vi "Modbus Master Example.vi"() -> ()   [LabVIEW 2013, in "Modbus Library - Advance.lvlib"]
doc: "An example of the modbus master functionality."
uses:
  Modbus Library - Advance.lvlib
  API/Wrapper/API Main.lvlib
  Master Function Definition/Read Device ID code.ctl
  Data Model/Device Data Model.lvclass
  API/Master/Modbus Master.lvclass
  API/Wrapper/Create TCP Master.vi
panel:
  in  "unit ID":u8=1
  in  "Stop Button":bool
  in  "Port":u16=502
  in  "Set Holding Registers":bool
  in  "Set Coils":bool
  in  "Fetch Discrete Inputs":bool
  in  "Fetch Input Registers":bool
  in  "Fetch Basic Objects":bool
  out "Basic Objects":string[](array[string])
  out "Status":string
  in  "Disconnect":bool
  in  "Connect":bool
  in  "Holding Registers":u16[](array[numeric])=[0, 0, 0, 0, 0, 0, 0, 0]
  out "Input Registers":u16[](array[numeric])
  in  "Coils":bool[](array[boolean])=[FALSE, FALSE, FALSE, FALSE, FALSE, FALSE, FALSE, FALSE]
  out "Discrete Inputs":bool[](array[boolean])
  in  "Slave Address":string="localhost"
  # "Coils are the boolean outputs of a modbus device. This example allows you to set the first 8 outputs."
  # "Holding Registers are the integer outputs of a modbus device. This example allows you to set the first 8 outputs."
  # "Modbus devices can also store objects in their memory, which are variable length strings. This example requests the basic level of objects."
  # "Discrete inputs are the boolean inputs of a modbus device. This example allows you to read the first 8 inputs."
  # "Input Registers are the integer inputs of a modbus device. This example allows you to read the first 8 inputs."
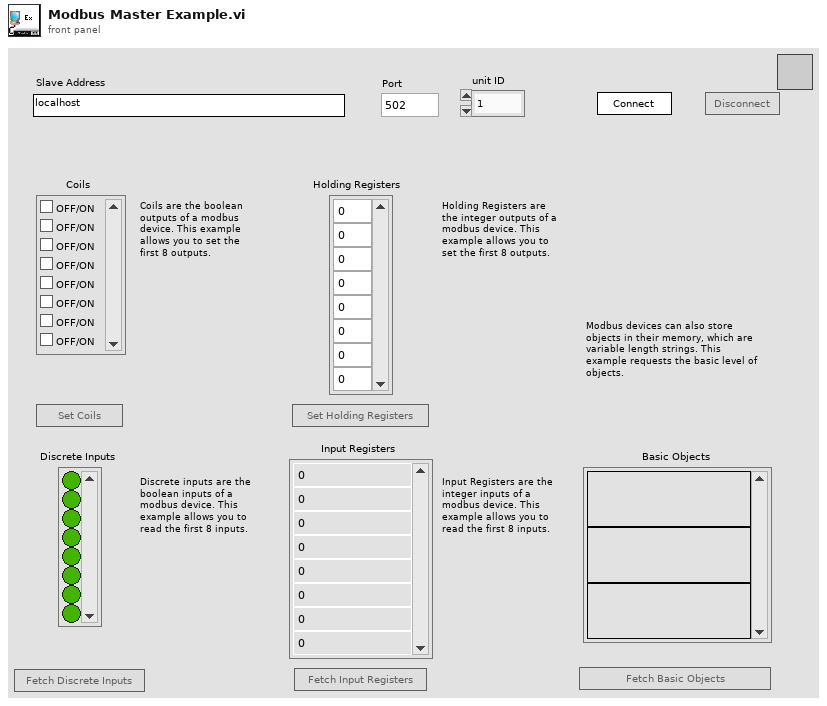
[diagram p1: front panel]
types:
  T1 = enum8{"Enabled", "Disabled", "Disabled and Grayed Out"}
  T2 = typedef "Modbus Library - Advance.lvlib/Device Data Model.lvclass/Read Device ID code.ctl" = enum8{"Read Basic", "Read Regular", "Read Extended", "Read Specific"}
  T3 = typedef "Modbus Library - Advance.lvlib/Device Data Model.lvclass/Identification Parameters.ctl" = cluster{"Object ID":u8, "Value":string}
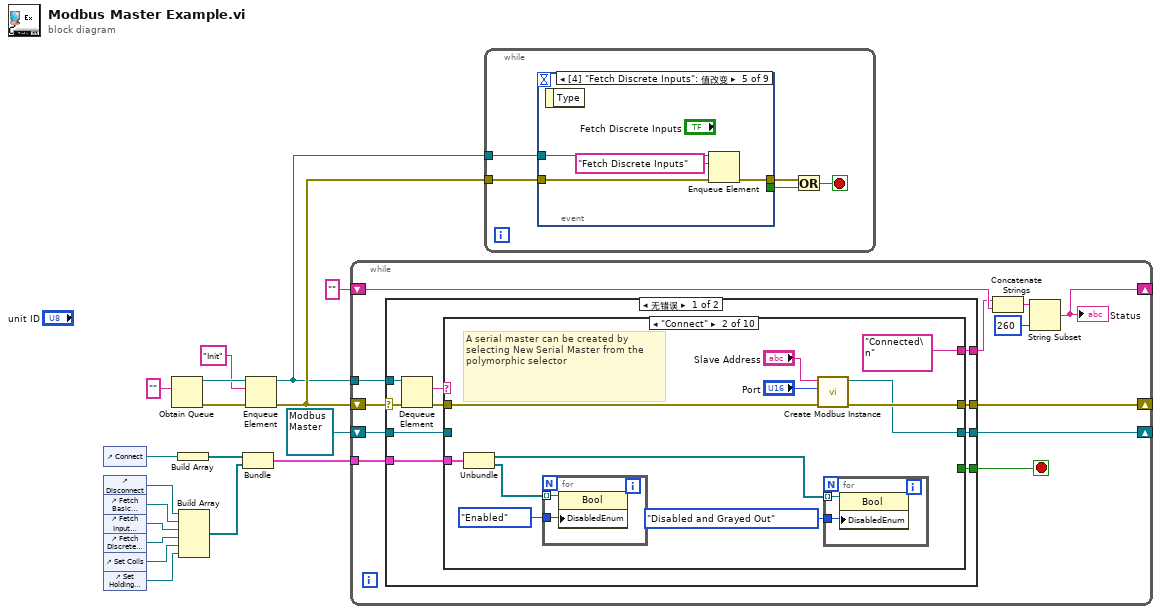
[diagram p0: block diagram]
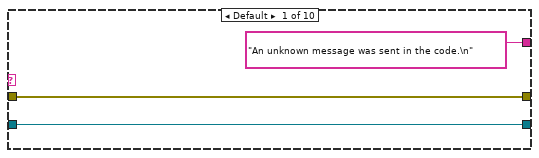
[diagram p2: hidden frame]
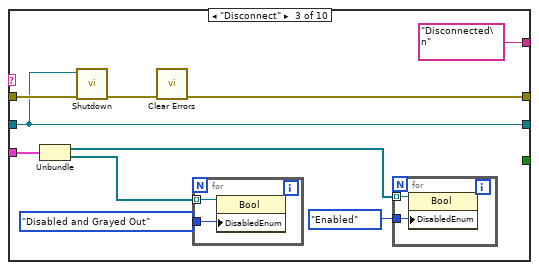
[diagram p3: hidden frame]
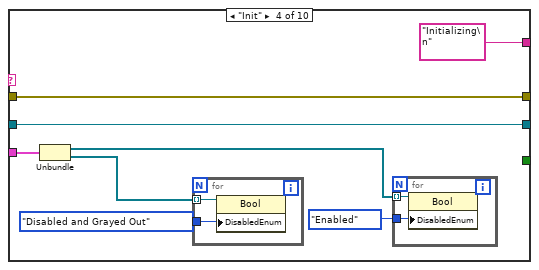
[diagram p4: hidden frame]
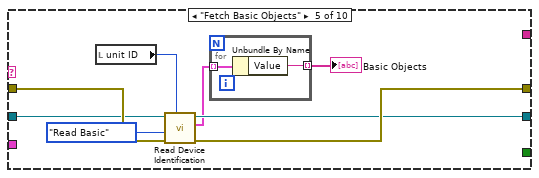
[diagram p5: hidden frame]
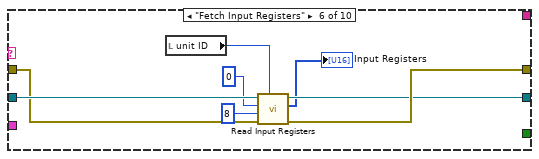
[diagram p6: hidden frame]
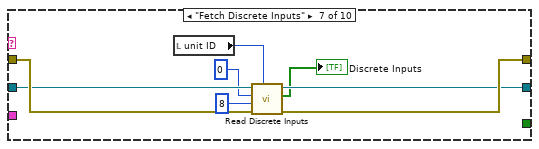
[diagram p7: hidden frame]
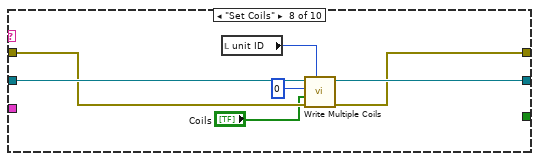
[diagram p8: hidden frame]
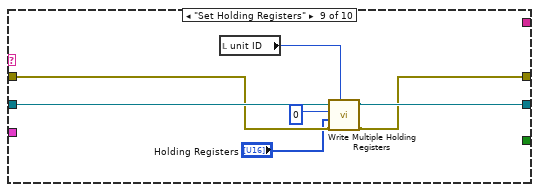
[diagram p9: hidden frame]
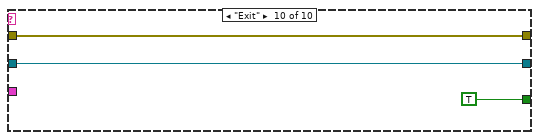
[diagram p10: hidden frame]
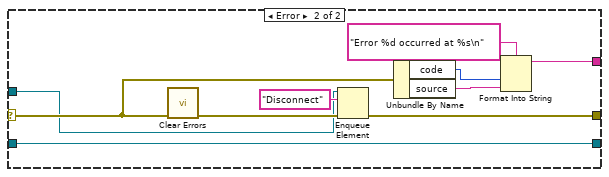
[diagram p11: hidden frame]
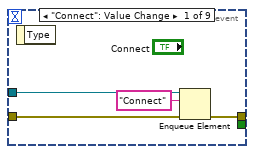
[diagram p12: hidden frame]
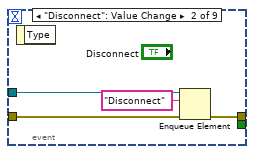
[diagram p13: hidden frame]
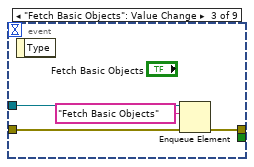
[diagram p14: hidden frame]
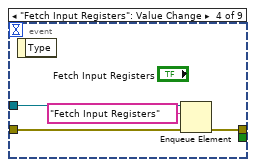
[diagram p15: hidden frame]
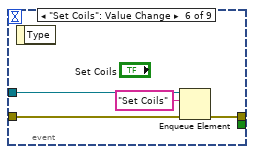
[diagram p16: hidden frame]
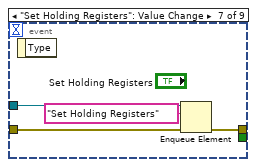
[diagram p17: hidden frame]
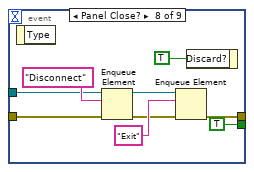
[diagram p18: hidden frame]
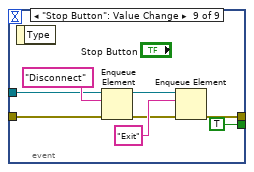
[diagram p19: hidden frame]
diagram:
  n1 = control-ref of="Connect"() -> (w9:refnum<vi>)
  n2 = control-ref of="Disconnect"() -> (w15:refnum<vi>)
  n3 = control-ref of="Fetch Basic Objects"() -> (w14:refnum<vi>)
  n4 = control-ref of="Fetch Input Registers"() -> (w13:refnum<vi>)
  n5 = control-ref of="Fetch Discrete Inputs"() -> (w12:refnum<vi>)
  n6 = control-ref of="Set Coils"() -> (w11:refnum<vi>)
  n7 = control-ref of="Set Holding Registers"() -> (w10:refnum<vi>)
  n8 = Obtain Queue(element data type="") -> (queue out=w4:refnum<queue>, error out=w18:errorcluster)  [unwired: 4 in, 1 out]
  n9 = Build Array(w9) -> (w6:refnum<vi>[])
  n10 = Build Array(w15, w14, w13, w12, w11, w10) -> (w8:refnum<vi>[])
  n11 = Bundle(w6, w8) -> (w7:cluster{refnum<vi>[], refnum<vi>[]})  [unwired: 1 in]
  n12 = Enqueue Element(queue=w4, element="Init", error in (no error)=w18) -> (queue out=w3:refnum<queue>, error out=w5:errorcluster)  [unwired: 1 in, 1 out]
  n13 = while {
    shift-right: [w22] -> _
    shift-left: refnum<class "Modbus Master.lvclass"> refnum ("Modbus Master") -> [w21]
    tunnel: w3 -> [w30]
    shift-right: [w28] -> _
    shift-left: w5 -> [w29]
    shift-right: [w27] -> _
    shift-left: "" ("Status") -> [w24]
    tunnel: w7 -> [w19]
    stop <- w20 stop-if-true
    n14 = case shown="无错误" w29 {
      selector: w29 -> [w39 w135]
      tunnel: w30 -> [w40 w129]
      tunnel: [w36 w136] -> w28
      tunnel: [w33 w132] -> w23
      tunnel: [w35 w128] -> w22
      tunnel: w21 -> [w34 w128]
      tunnel: [w32 _] -> w20
      tunnel: w19 -> [w31 _]
      frame No Error {
        n15 = Dequeue Element(queue=w40, error in (no error)=w39) -> (element=w37:string, error out=w38:errorcluster)  [unwired: 1 in, 2 out]
        n16 = case shown="\"Connect\"" w37 {
          tunnel: w38 -> [w43 w53 w68 w80 w92 w99 w110 w114 w121 w127]
          tunnel: [w43 w52 w64 w80 w91 w102 w109 w115 w122 w127] -> w36
          tunnel: [w42 w51 w66 w79 w89 w101 w107 w116 w123 w126] -> w35
          tunnel: w34 -> [w42 _ w66 w79 w90 w100 w108 w117 w124 w126]
          tunnel: ["An unknown message was sent in the code.\n" "Connected\n" "Disconnected\n" "Initializing\n" _ _ _ _ _ _] -> w33
          tunnel: [_ _ _ _ _ _ _ _ _ TRUE] -> w32
          tunnel: w31 -> [_ w49 w63 w77 _ _ _ _ _ _]
          frame Default {
          }
          frame "Connect" {
            # "A serial master can be created by selecting New Serial Master from the polymorphic selector"
            n17 = Unbundle(w49) -> (w47:refnum<vi>[], w48:refnum<vi>[])
            n18 = for {
              tunnel: w48 -> [w56] mode=indexing
              tunnel: T1."Enabled" ("Disabled") -> [w55]
              n19 = property class="Bool"(reference=w56, "DisabledEnum"=w55) -> ()  [unwired: 1 in, 2 out]
            }
            n20 = call-poly "Create Modbus Instance.vi"("error in"=w53, "port (502)"="Port", "address"="Slave Address") -> ("error out"=w52:errorcluster, "TCP master instance"=w51:refnum<class "Modbus Master.lvclass">)  [unwired: 7 in]
            n21 = for {
              tunnel: w47 -> [w58] mode=indexing
              tunnel: T1."Disabled and Grayed Out" ("Disabled") -> [w57]
              n22 = property class="Bool"(reference=w58, "DisabledEnum"=w57) -> ()  [unwired: 1 in, 2 out]
            }
          }
          frame "Disconnect" {
            n23 = Unbundle(w63) -> (w61:refnum<vi>[], w62:refnum<vi>[])
            n24 = call-dynamic "Shutdown.vi"("error in"=w68, "Modbus master in"=w66) -> ("error out"=w67:errorcluster)  [unwired: 9 in]
            n25 = call <vilib>:"Clear Errors.vi"("error in (no error)"=w67) -> ("error out"=w64:errorcluster)  [unwired: 6 in]
            n26 = for {
              tunnel: w62 -> [w72] mode=indexing
              tunnel: T1."Disabled and Grayed Out" ("Disabled") -> [w71]
              n27 = property class="Bool"(reference=w72, "DisabledEnum"=w71) -> ()  [unwired: 1 in, 2 out]
            }
            n28 = for {
              tunnel: w61 -> [w70] mode=indexing
              tunnel: T1."Enabled" ("Disabled") -> [w69]
              n29 = property class="Bool"(reference=w70, "DisabledEnum"=w69) -> ()  [unwired: 1 in, 2 out]
            }
          }
          frame "Init" {
            n30 = Unbundle(w77) -> (w75:refnum<vi>[], w76:refnum<vi>[])
            n31 = for {
              tunnel: w76 -> [w84] mode=indexing
              tunnel: T1."Disabled and Grayed Out" ("Disabled") -> [w83]
              n32 = property class="Bool"(reference=w84, "DisabledEnum"=w83) -> ()  [unwired: 1 in, 2 out]
            }
            n33 = for {
              tunnel: w75 -> [w82] mode=indexing
              tunnel: T1."Enabled" ("Disabled") -> [w81]
              n34 = property class="Bool"(reference=w82, "DisabledEnum"=w81) -> ()  [unwired: 1 in, 2 out]
            }
          }
          frame "Fetch Basic Objects" {
            n35 = local read "unit ID"() -> (w85:u8)
            n36 = call-dynamic "Read Device Identification.vi"("unit ID"=w85, "error in"=w92, "read device ID code"=Read_Device_ID_code."Read Basic" ("Read Device ID code"), "Modbus master in"=w90) -> ("error out"=w91:errorcluster, "objects"=w87:T3[], "Modbus master out"=w89:refnum<class "Modbus Master.lvclass">)  [unwired: 5 in]
            n37 = for {
              tunnel: w87 -> [w94] mode=indexing
              tunnel: [w93] -> w86 mode=indexing
              n38 = Unbundle By Name(w94) -> ("Value"=w93:string)
            }
            "Basic Objects" <- w86
          }
          frame "Fetch Input Registers" {
            n39 = local read "unit ID"() -> (w95:u8)
            n40 = call-dynamic "Read Input Registers.vi"("unit ID"=w95, "error in"=w99, "number of inputs"=u16 8 ("number of registers"), "starting address"=u16 0, "Modbus master in"=w100) -> ("error out"=w102:errorcluster, "register values"=→"Input Registers":u16[], "Modbus master out"=w101:refnum<class "Modbus Master.lvclass">)  [unwired: 4 in]
          }
          frame "Fetch Discrete Inputs" {
            n41 = local read "unit ID"() -> (w103:u8)
            n42 = call-dynamic "Read Discrete Inputs.vi"("unit ID"=w103, "error in"=w110, "number of inputs"=u16 8, "starting address"=u16 0, "Modbus master in"=w108) -> ("error out"=w109:errorcluster, "discrete inputs"=→"Discrete Inputs":bool[], "Modbus master out"=w107:refnum<class "Modbus Master.lvclass">)  [unwired: 4 in]
          }
          frame "Set Coils" {
            n43 = local read "unit ID"() -> (w111:u8)
            n44 = call-dynamic "Write Multiple Coils.vi"("unit ID"=w111, "error in"=w114, "coils to write"="Coils", "starting address"=u16 0, "Modbus master in"=w117) -> ("error out"=w115:errorcluster, "Modbus master out"=w116:refnum<class "Modbus Master.lvclass">)  [unwired: 5 in]
          }
          frame "Set Holding Registers" {
            n45 = local read "unit ID"() -> (w118:u8)
            n46 = call-dynamic "Write Multiple Holding Registers.vi"("unit ID"=w118, "error in"=w121, "registers to write"="Holding Registers", "starting address"=u16 0, "Modbus master in"=w124) -> ("error out"=w122:errorcluster, "Modbus master out"=w123:refnum<class "Modbus Master.lvclass">)  [unwired: 5 in]
          }
          frame "Exit" {
          }
        }
      }
      frame Error {
        n47 = call <vilib>:"Clear Errors.vi"("error in (no error)"=w135) -> ("error out"=w137:errorcluster)  [unwired: 6 in]
        n48 = Enqueue Element(queue=w129, element="Disconnect", error in (no error)=w137) -> (error out=w136:errorcluster)  [unwired: 1 in, 2 out]
        n49 = Unbundle By Name(w135) -> ("code"=w134:i32, "source"=w133:string)
        n50 = Format Into String(format string="Error %d occurred at %s\n", w134, w133) -> (resulting string=w132:string)  [unwired: 2 in, 1 out]
      }
    }
    n51 = Concatenate Strings(w23, w24) -> (w25:string)
    n52 = String Subset(string=w25, length (rest)=260 ("length (rest)")) -> (substring=w27:string)  [unwired: 1 in]
    "Status" <- w27
  }
  n53 = while {
    tunnel: w5 -> [w142]
    tunnel: w3 -> [w141]
    stop <- w138 stop-if-true
    n54 = event shown="[4] \"Fetch Discrete Inputs\": 值改变" {
      selector: _ -> [_ _ _ _ _ _ _ _ _]
      dyn-events: _ -> [_ _ _ _ _ _ _ _ _]
      timeout: _ -> [_ _ _ _ _ _ _ _ _]
      tunnel: w142 -> [w146 w150 w154 w158 w162 w166 w170 w176 w185]
      tunnel: [w145 w149 w153 w157 w161 w165 w169 w171 w180] -> w140
      tunnel: w141 -> [w144 w148 w152 w156 w160 w164 w168 w173 w182]
      tunnel: [_ _ _ _ _ _ _ TRUE ("Discard?") TRUE ("Discard?")] -> w139
      event "Connect": Value Change {
        n55 = event-data() -> ()  [unwired: 1 in, 1 out]
        n56 = Enqueue Element(queue=w144, element="Connect", error in (no error)=w146) -> (error out=w145:errorcluster)  [unwired: 1 in, 2 out]
      }
      event "Disconnect": Value Change {
        n57 = event-data() -> ()  [unwired: 1 in, 1 out]
        n58 = Enqueue Element(queue=w148, element="Disconnect", error in (no error)=w150) -> (error out=w149:errorcluster)  [unwired: 1 in, 2 out]
      }
      event "Fetch Basic Objects": Value Change {
        n59 = event-data() -> ()  [unwired: 1 in, 1 out]
        n60 = Enqueue Element(queue=w152, element="Fetch Basic Objects", error in (no error)=w154) -> (error out=w153:errorcluster)  [unwired: 1 in, 2 out]
      }
      event "Fetch Input Registers": Value Change {
        n61 = event-data() -> ()  [unwired: 1 in, 1 out]
        n62 = Enqueue Element(queue=w156, element="Fetch Input Registers", error in (no error)=w158) -> (error out=w157:errorcluster)  [unwired: 1 in, 2 out]
      }
      event "Fetch Discrete Inputs": Value Change {
        n63 = event-data() -> ()  [unwired: 1 in, 1 out]
        n64 = Enqueue Element(queue=w160, element="Fetch Discrete Inputs", error in (no error)=w162) -> (error out=w161:errorcluster)  [unwired: 1 in, 2 out]
      }
      event "Set Coils": Value Change {
        n65 = event-data() -> ()  [unwired: 1 in, 1 out]
        n66 = Enqueue Element(queue=w164, element="Set Coils", error in (no error)=w166) -> (error out=w165:errorcluster)  [unwired: 1 in, 2 out]
      }
      event "Set Holding Registers": Value Change {
        n67 = event-data() -> ()  [unwired: 1 in, 1 out]
        n68 = Enqueue Element(queue=w168, element="Set Holding Registers", error in (no error)=w170) -> (error out=w169:errorcluster)  [unwired: 1 in, 2 out]
      }
      event Panel Close? {
        n69 = event-data() -> ()  [unwired: 1 in, 1 out]
        n70 = Enqueue Element(queue=w173, element="Disconnect", error in (no error)=w176) -> (queue out=w174:refnum<queue>, error out=w172:errorcluster)  [unwired: 1 in, 1 out]
        n71 = Enqueue Element(queue=w174, element="Exit", error in (no error)=w172) -> (error out=w171:errorcluster)  [unwired: 1 in, 2 out]
        n72 = event-data("Discard?"=TRUE) -> ()  [unwired: 1 in, 1 out]
      }
      event "Stop Button": Value Change {
        n73 = event-data() -> ()  [unwired: 1 in, 1 out]
        n74 = Enqueue Element(queue=w182, element="Disconnect", error in (no error)=w185) -> (queue out=w183:refnum<queue>, error out=w181:errorcluster)  [unwired: 1 in, 1 out]
        n75 = Enqueue Element(queue=w183, element="Exit", error in (no error)=w181) -> (error out=w180:errorcluster)  [unwired: 1 in, 2 out]
      }
    }
    n76 = Or(x=w140, y=w139) -> (x .or. y?=w138:bool)
  }
